vi "LV SciSDK INIT DIGITIZER.vi"(0 "Digitizer Name":string, 1 "Acq mode":string(combo)="blocking", 2 "Timeout":i32=100, 3 "High performance":string(combo)="false", 5 "Enabled channels":u32=1, 7 "Acq len":u32=1024, 9 "Handle In":T2, 11 "error in (no error)":errorcluster) -> (10 "Digitizer Handle Out":T1, 15 "error out":errorcluster)   [LabVIEW 2021]
uses:
  SciSDK_Labview.lvlib
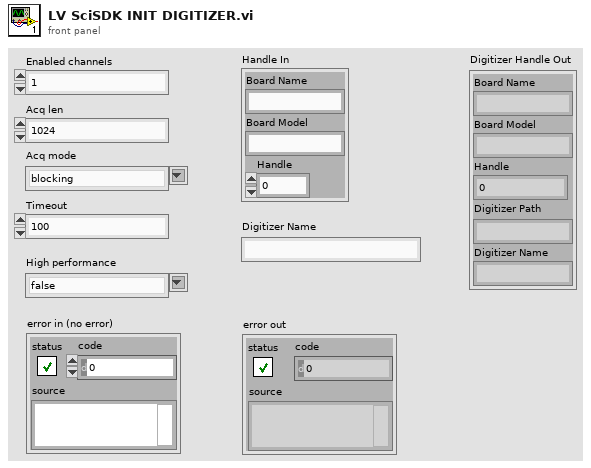
[diagram p1: front panel]
types:
  T1 = cluster{"Board Name":string, "Board Model":string, "Handle":u64, "Digitizer Path":string, "Digitizer Name":string}
  T2 = cluster{"Board Name":string, "Board Model":string, "Handle":u64}
  T3 = cluster{"Board Name":string, "Board Model":string, "Handle":u64, string, "Digitizer Name":string}
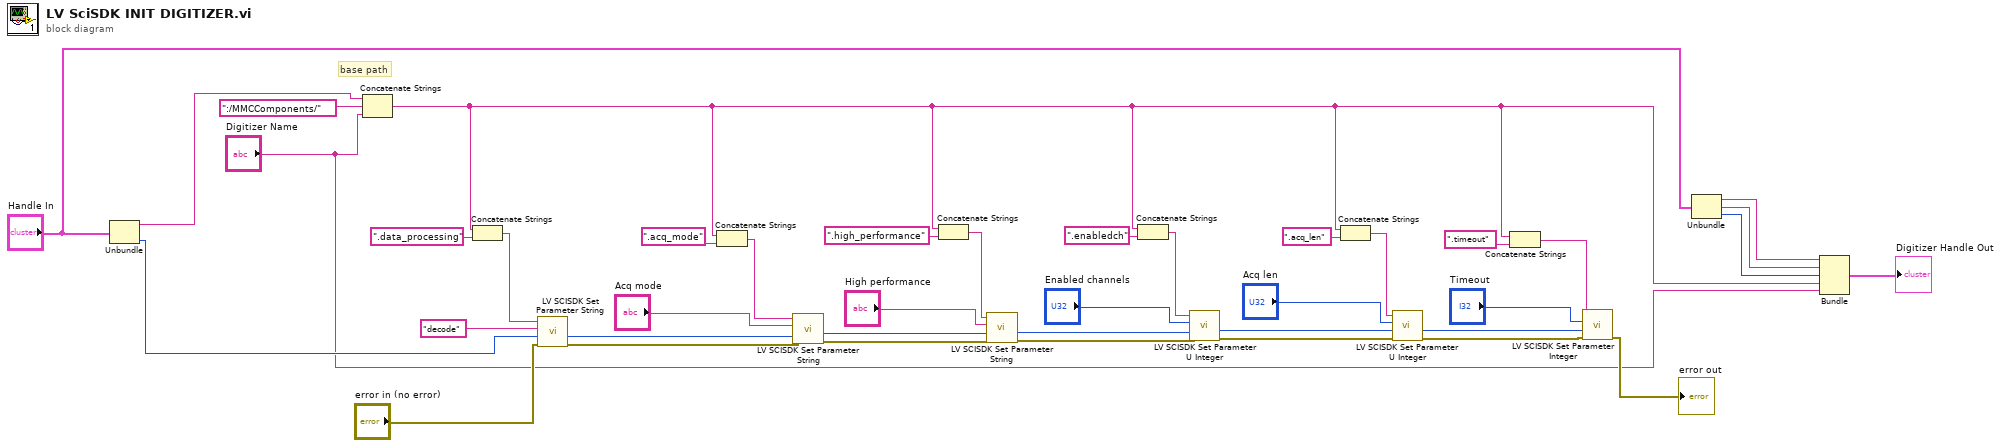
[diagram p0: block diagram]
diagram:
  # "base path"
  n1 = Unbundle("Handle In") -> ("Board Name"=w39:string, "Handle"=w35:u64)  [unwired: 1 out]
  n2 = Concatenate Strings(w39, ":/MMCComponents/" ("string"), "Digitizer Name") -> (w3:string)
  n3 = Concatenate Strings(w3, ".data_processing" ("string")) -> (w37:string)
  n4 = call "LV SCISDK Set Parameter String.vi"("error in (no error)"="error in (no error)", "handle"=w35, "value"="decode", "Path"=w37) -> ("error out"=w33:errorcluster, "handle out"=w24:u64)  [unwired: 5 in, 1 out]
  n5 = Concatenate Strings(w3, ".acq_mode" ("string")) -> (w26:string)
  n6 = call "LV SCISDK Set Parameter String.vi"("error in (no error)"=w33, "handle"=w24, "value"="Acq mode", "Path"=w26) -> ("error out"=w32:errorcluster, "handle out"=w23:u64)  [unwired: 5 in, 1 out]
  n7 = Concatenate Strings(w3, ".high_performance" ("string")) -> (w21:string)
  n8 = call "LV SCISDK Set Parameter String.vi"("error in (no error)"=w32, "handle"=w23, "value"="High performance", "Path"=w21) -> ("error out"=w20:errorcluster, "handle out"=w19:u64)  [unwired: 5 in, 1 out]
  n9 = Concatenate Strings(w3, ".enabledch" ("string")) -> (w18:string)
  n10 = call "LV SCISDK Set Parameter U Integer.vi"("error in (no error)"=w20, "handle"=w19, "value"="Enabled channels", "Path"=w18) -> ("error out"=w16:errorcluster, "handle out"=w15:u64)  [unwired: 5 in, 1 out]
  n11 = Concatenate Strings(w3, ".acq_len" ("string")) -> (w13:string)
  n12 = call "LV SCISDK Set Parameter U Integer.vi"("error in (no error)"=w16, "handle"=w15, "value"="Acq len", "Path"=w13) -> ("error out"=w12:errorcluster, "handle out"=w10:u64)  [unwired: 5 in, 1 out]
  n13 = Concatenate Strings(w3, ".timeout" ("string")) -> (w9:string)
  n14 = call "LV SCISDK Set Parameter Integer.vi"("error in (no error)"=w12, "handle"=w10, "value"="Timeout", "Path"=w9) -> ("error out"=→"error out":errorcluster)  [unwired: 5 in, 2 out]
  n15 = Unbundle("Handle In") -> ("Board Name"=w7:string, "Board Model"=w6:string, "Handle"=w5:u64)
  n16 = Bundle("Board Name"=w7, "Board Model"=w6, "Handle"=w5, w3, "Digitizer Name"="Digitizer Name") -> (→"Digitizer Handle Out":T3)  [unwired: 1 in]
